vi "Init.vi"(8 "error in (no error)":errorcluster caption="entrée d'erreur (pas d'erreur)", 11 "Class UART (Default) en entrée":refnum<class "Class UART Enocean.lvclass">) -> (0 "error out":errorcluster caption="sortie d'erreur", 3 "Class UART (Default) en sortie":refnum<class "Class UART Enocean.lvclass">)   [LabVIEW 2020, in "Library Instrument & Equipement.lvlib" / "Library UART.lvlib" / "Class UART Enocean.lvclass"]
uses:
  Class UART Enocean.lvclass
  C:/Users/ngarcin/OneDrive - Altyor/Standard TB/Class/UART/UART (Default)/Class UART (Default).lvclass
  UART (Default)/Class UART (Default).lvclass
  Class UART Enocean.lvclass/Class UART Enocean.ctl
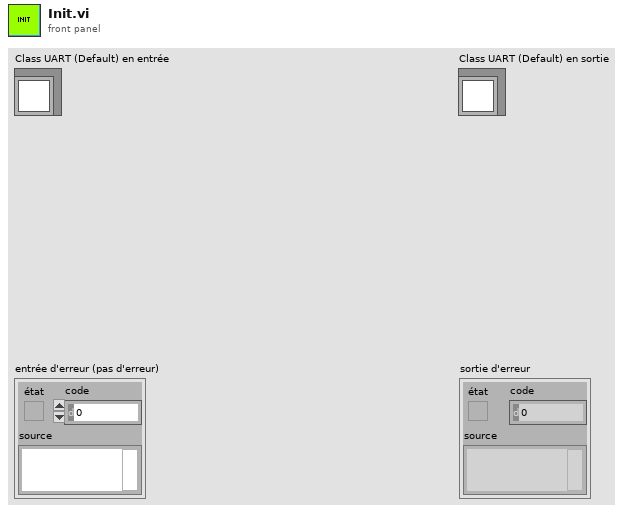
[diagram p1: front panel]
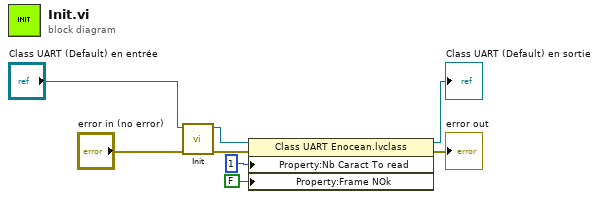
[diagram p0: block diagram]
diagram:
  n1 = call-parent "Init.vi"("error in (no error)"="error in (no error)", "Class UART (Default) en entrée"="Class UART (Default) en entrée") -> ("error out"=w5:errorcluster, "Class UART (Default) en sortie"=w4:refnum<class "Class UART Enocean.lvclass">)  [unwired: 8 in]
  n2 = property class="Class UART Enocean.lvclass"(reference=w4, error in=w5, "Property:Nb Caract To read"=u32 1 ("Nb Caract To read"), "Property:Frame NOk"=FALSE ("Frame NOk")) -> (reference out=→"Class UART (Default) en sortie":refnum<class "Class UART Enocean.lvclass">, error out=→"error out":errorcluster)
